vi "Assign_Label_and_Answer.vi"(6 "Start in":i32, 9 "Stop in":i32, 10 "Array in":sgl[][](array[numeric]), 11 "Trial Flag":bool) -> (1 "Start out":i32, 2 "Stop out":i32, 3 "Array out":sgl[][](array[numeric]))   [LabVIEW 2020]
uses:
  Global Variables/Global User_Answer.vi
  Global Variables/Global Label.vi
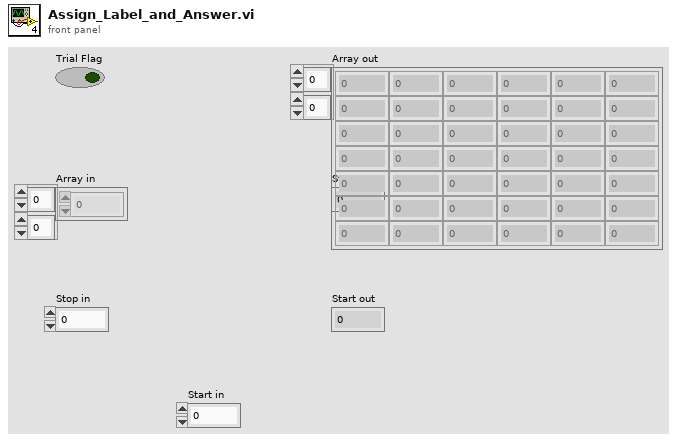
[diagram p1: front panel]
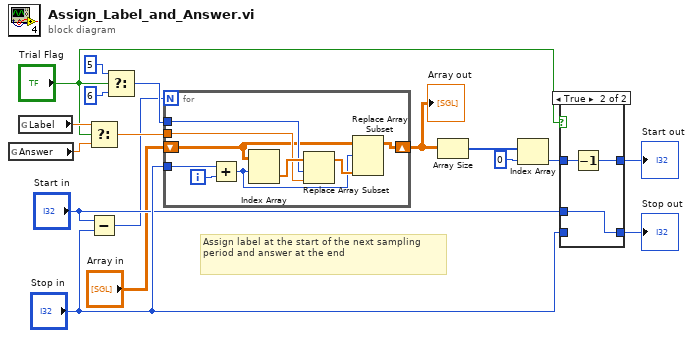
[diagram p0: block diagram]
diagram:
  # "Assign label at the start of the next sampling period and answer at the end"
  n1 = global read "Global User_Answer.vi" "Answer"() -> (w6:dbl)
  n2 = global read "Global Label.vi" "Label"() -> (w5:dbl)
  n3 = Select(t=w5, s="Trial Flag", f=w6) -> (s? t:f=w14:dbl)
  n4 = Subtract(x="Start in", y="Stop in") -> (x-y=w4:i32)
  n5 = Select(t=5, s="Trial Flag", f=6) -> (s? t:f=w15:i32)
  n6 = for {
    N: w4 -> [_]
    tunnel: "Stop in" -> [w26]
    shift-right: [w18] -> w3
    shift-left: "Array in" -> [w21]
    tunnel: w14 -> [w23]
    tunnel: w15 -> [w22]
    i -> [w25]
    n7 = Add(x=w26, y=w25) -> (x+y=w19:i32)
    n8 = Index Array(array=w21, index (row)=w19) -> (element=w24:sgl[])  [unwired: 1 in]
    n9 = Replace Array Subset(array=w24, new element=w23, index=w22) -> (w20:sgl[])
    n10 = Replace Array Subset(array=w21, new element=w20, index (row)=w19) -> (w18:sgl[][])  [unwired: 1 in]
  }
  "Array out" <- w3
  n11 = Array Size(array=w3) -> (size(s)=w12:i32[])
  n12 = Index Array(array=w12, index=0) -> (element=w11:i32)
  n13 = case shown="True" "Trial Flag" {
    tunnel: "Start in" -> [w28 w29]
    tunnel: [w28 w31] -> w8
    tunnel: [w27 w29] -> w10
    tunnel: "Stop in" -> [w27 _]
    tunnel: w11 -> [_ w30]
    frame False {
    }
    frame True {
      n14 = Decrement(x=w30) -> (x-1=w31:i32)
    }
  }
  "Stop out" <- w10
  "Start out" <- w8
